vi "生成所有扫描曲线.vi"(8 "簇输入":cluster{"数据":T1[], "显示数据":i32[]}, 10 "曲线设置":T3, 11 "坐标轴映射":T4) -> (0 "簇输出":cluster{"数据":T1[], "显示数据":i32[]}, 3 "曲线":cluster{dbl[], dbl[]}[](array[cluster]))   [LabVIEW 2021]
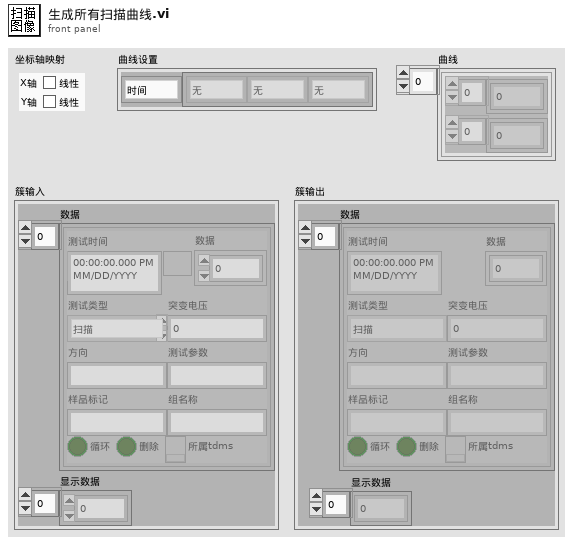
[diagram p1: front panel]
types:
  T1 = typedef "测试数据类型.ctl" = cluster{"测试时间":timestamp, "测试类型":T2, "方向":string, "样品标记":string, "测试参数":string, "循环":bool, "删除":bool, "组名称":string, "所属tdms":refnum<k34>, "突变电压":i32, "数据":dbl[][]}
  T2 = typedef "测试类型.ctl" = enum16{"扫描", "脉冲", "维持时间"}
  T3 = typedef "曲线设置.ctl" = cluster{"X轴数据选择":enum16{"时间", "设置电压", "读取电流", "读取电压"}, "Y轴组":enum16{"时间", "设置电压", "读取电流", "读取电压", "无"}[]}
  T4 = typedef "坐标轴映射.ctl" = cluster{"X轴":bool, "Y轴":bool}
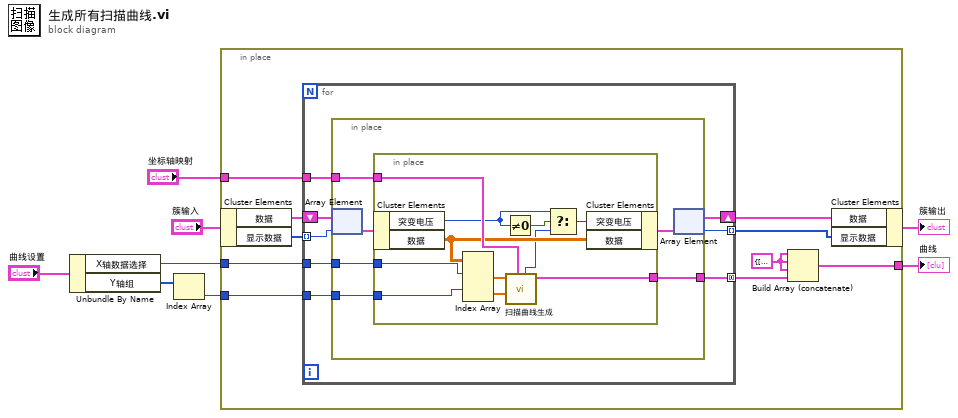
[diagram p0: block diagram]
diagram:
  n1 = Unbundle By Name("曲线设置") -> ("X轴数据选择"=w3:enum16{"时间", "设置电压", "读取电流", "读取电压"}, "Y轴组"=w4:enum16{"时间", "设置电压", "读取电流", "读取电压", "无"}[])
  n2 = Index Array(array=w4) -> (element=w2:enum16{"时间", "设置电压", "读取电流", "读取电压", "无"})  [unwired: 1 in]
  n3 = in-place {
    in-place-border: "坐标轴映射" -> [w18]
    in-place-border: [w13] -> w7
    in-place-border: w3 -> [w12]
    in-place-border: w2 -> [w11]
    w9 = cluster{dbl[], dbl[]} {[0.0], [0.0]}
    n4 = in-place-cluster #1("簇输入") -> ("数据"=w17:T1[], "显示数据"=w14:i32[])
    n5 = for {
      tunnel: w18 -> [w26]
      tunnel: [w25] -> w10 mode=concatenating
      tunnel: w14 -> [w23] mode=indexing
      tunnel: [w21] -> w15 mode=indexing
      shift-right: [w22] -> w16
      shift-left: w17 -> [w24]
      tunnel: w12 -> [w20]
      tunnel: w11 -> [w19]
      n6 = in-place {
        in-place-border: w26 -> [w32]
        in-place-border: [w31] -> w25
        in-place-border: w20 -> [w28]
        in-place-border: w19 -> [w27]
        n7 = in-place-array #2(w24, w23) -> (w30:T1)
        n8 = in-place {
          in-place-border: w32 -> [w43]
          in-place-border: [w40] -> w31
          in-place-border: w28 -> [w34]
          in-place-border: w27 -> [w33]
          n9 = in-place-cluster #3(w30) -> ("突变电压"=w36:i32, "数据"=w39:dbl[][])
          n10 = Index Array(array=w39, index (row) #1=w34, index (row) #2=w33) -> (element #1=w42:dbl[], element #2=w41:dbl[])  [unwired: 2 in]
          n11 = Not Equal To 0?(x=w36) -> (x != 0?=w38:bool)
          n12 = call "扫描曲线生成.vi"("坐标轴映射"=w43, "Y"=w41, "X"=w42) -> ("曲线"=w40:cluster{dbl[], dbl[]}[], "突变电压"=w37:i32)  [unwired: 7 in]
          n13 = Select(t=w36, s=w38, f=w37) -> (s? t:f=w35:i32)
          n14 = in-place-cluster #3("突变电压"=w35, "数据"=w39) -> (w29:T1)
        }
        n15 = in-place-array #2(w29) -> (w22:T1[], w21:i32)
      }
    }
    n16 = Build Array (concatenate)(w9, w9, w9, w10) -> (w13:cluster{dbl[], dbl[]}[])
    n17 = in-place-cluster #1("数据"=w16, "显示数据"=w15) -> (→"簇输出":cluster{"数据":T1[], "显示数据":i32[]})
  }
  "曲线" <- w7
